vi "Lorentzian complex model.vi"() -> ()   [LabVIEW 2016]
uses:
  <vilib>/Analysis/NI_AAL_SigProc.lvlib
  <vilib>/Analysis/NI_AALBase.lvlib
panel:
  out "Gama guess":dbl
  out "2nd Derivatives":dbl[](array[numeric])
  out "Amplitudes":dbl[](array[numeric])
  out "Locations":dbl[](array[numeric])
  out "Waveform Graph 2":dbl[](graph)
  out "standard deviation":dbl format="%0.2f"
  out "Circle plot":cluster{dbl[], dbl[]}(graph)
  in  "phase":dbl
  in  "Amplitude":dbl=50.0
  in  "Range":i32=100
  in  "Gamma":dbl=10.0
  in  "F0":i32=50
  out "Waveform Graph":dbl[][](graph)
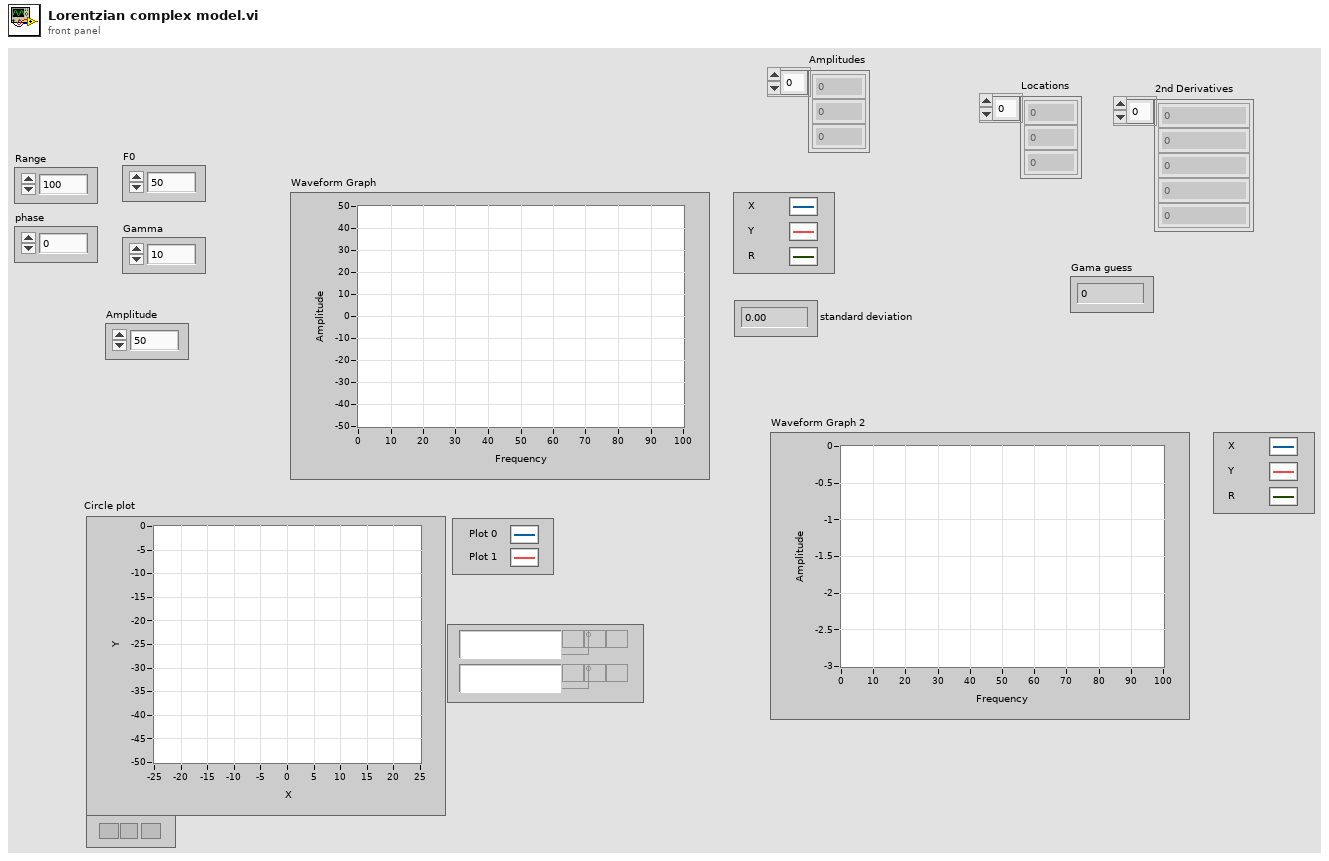
[diagram p1: front panel]
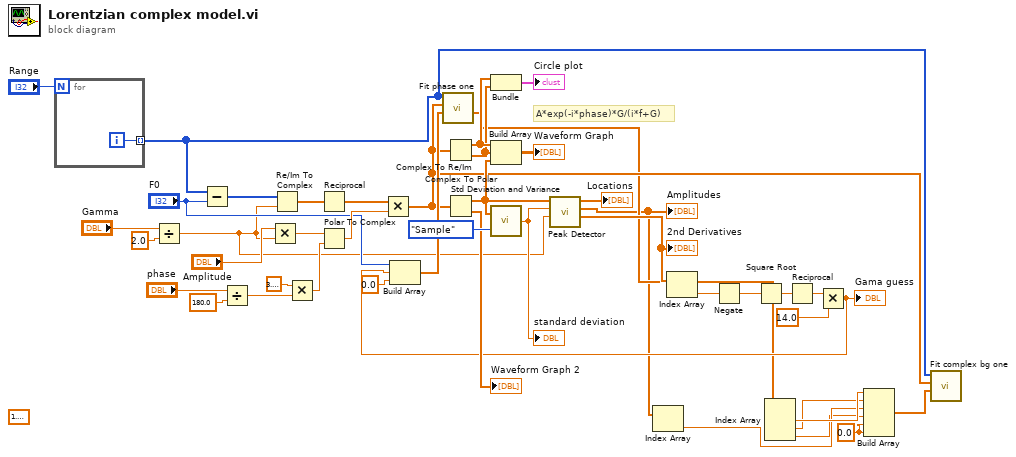
[diagram p0: block diagram]
diagram:
  w1 = 0.0 ("element")
  (unwired) 1.5707963267948966
  # "A*exp(-i*phase)*G/(i*f+G)"
  n1 = for {
    N: "Range" -> [_]
    tunnel: [w45] -> w10 mode=indexing
    i -> [w45]
  }
  n2 = Divide(x="Gamma", y=2.0) -> (x/y=w12:dbl)
  n3 = Subtract(x=w10, y="F0") -> (x-y=w26:i32[])
  n4 = Divide(x="phase", y=180.0) -> (x/y=w37:dbl)
  n5 = Multiply(x="Amplitude", y=w12) -> (x*y=w27:dbl)
  n6 = Re/Im To Complex(1:w12, 2:w26) -> (0:w43:cdb[])
  n7 = Multiply(x=3.141592653589793, y=w37) -> (x*y=w35:dbl)
  n8 = Reciprocal(x=w43) -> (1/x=w42:cdb[])
  n9 = Polar To Complex(1:w35, 2:w27) -> (0:w38:cdb)
  n10 = Multiply(x=w42, y=w38) -> (x*y=w9:cdb[])
  n11 = Complex To Re/Im(x + iy=w9) -> (x=w33:dbl[], y=w32:dbl[])
  n12 = Complex To Polar(r * e^(i*theta)=w9) -> (r=w30:dbl[], theta=→"Waveform Graph 2":dbl[])
  n13 = Bundle(w33, w32) -> (→"Circle plot":cluster{dbl[], dbl[]})  [unwired: 1 in]
  n14 = Build Array(w33, w32, w30) -> (→"Waveform Graph":dbl[][])
  n15 = call <vilib>:"Std Deviation and Variance.vi"("X"=w30, "Weighting (Sample)"=enum16{"Sample", "Population"}."Sample") -> ("standard deviation"=w28:dbl)  [unwired: 2 out]
  "standard deviation" <- w28
  n16 = call <vilib>:"Peak Detector.vi"("width"=w12, "threshold"=w28, "X"=w30) -> ("2nd Derivatives"=w19:dbl[], "Amplitudes"=w4:dbl[], "Locations"=→"Locations":dbl[])  [unwired: 4 in, 2 out]
  "Amplitudes" <- w4
  "2nd Derivatives" <- w19
  n17 = Index Array(array=w4) -> (element=w3:dbl)  [unwired: 1 in]
  n18 = Index Array(array=w19) -> (element=w18:dbl)  [unwired: 1 in]
  n19 = Negate(x=w18) -> (-x=w17:dbl)
  n20 = Square Root(x=w17) -> (sqrt(x)=w16:dbl)
  n21 = Reciprocal(x=w16) -> (1/x=w15:dbl)
  n22 = Multiply(x=w15, y=14.0) -> (x*y=w11:dbl)
  "Gama guess" <- w11
  n23 = Build Array("F0", w11, 0.0 ("element")) -> (w22:dbl[])
  n24 = call "Fit phase one.vi"("Initial parameters"=w22, "Z"=w9, "X"=w10) -> ("best fit parameters"=w7:dbl[])  [unwired: 8 in]
  n25 = Index Array(array=w7) -> (element #1=w6:dbl, element #2=w5:dbl, element #3=w2:dbl)  [unwired: 3 in]
  n26 = Build Array(w6, w5, w3, w2, w1, w1) -> (w8:dbl[])
  n27 = call "Fit complex bg one.vi"("Initial parameters"=w8, "Z"=w9, "X"=w10) -> ()  [unwired: 9 in]
